vi "intepret.vi"(8 "error in (no error)":errorcluster, 10 "context":string, 11 "AndExpression in":refnum<class "AndExpression.lvclass">) -> (0 "error out":errorcluster, 2 "result":bool, 3 "AndExpression out":refnum<class "AndExpression.lvclass">)   [LabVIEW 2018, in "AndExpression.lvclass"]
uses:
  AndExpression.lvclass
  AndExpression.lvclass/AndExpression.ctl
  TerminalExpression Class/TerminalExpression.lvclass
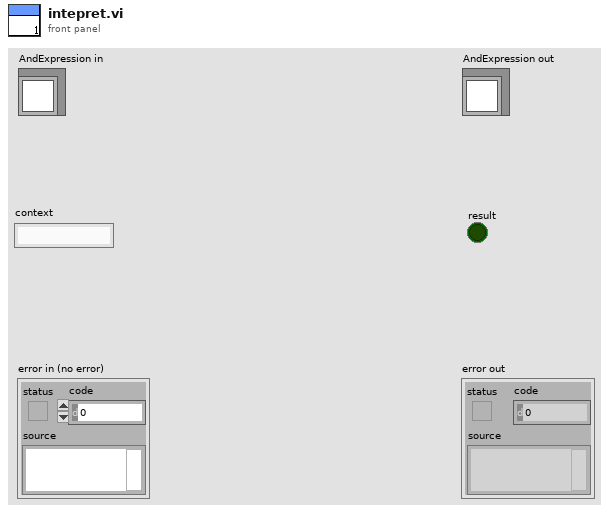
[diagram p1: front panel]
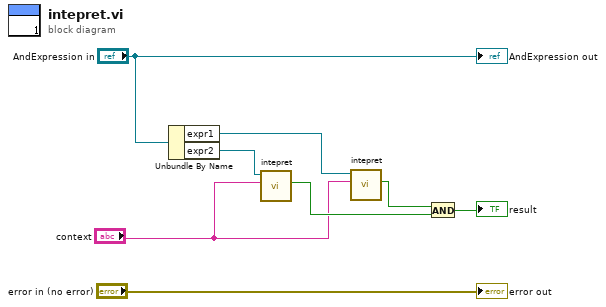
[diagram p0: block diagram]
diagram:
  n1 = Unbundle By Name("AndExpression in") -> ("expr1"=w6:refnum<class "TerminalExpression.lvclass">, "expr2"=w7:refnum<class "TerminalExpression.lvclass">)
  n2 = call-dynamic "intepret.vi"("context"="context", "TerminalExpression in"=w7) -> ("result"=w4:bool)  [unwired: 7 in, 2 out]
  n3 = call-dynamic "intepret.vi"("context"="context", "TerminalExpression in"=w6) -> ("result"=w5:bool)  [unwired: 7 in, 2 out]
  n4 = And(x=w5, y=w4) -> (x .and. y?=→"result":bool)
  "error out" <- "error in (no error)"
  "AndExpression out" <- "AndExpression in"
